vi "Mem_exper.vi"() -> ()   [LabVIEW 2018]
uses:
  <vilib>/Platform/TimedLoop/XDataNode/timing_clust.ctl
  <vilib>/Platform/TimedLoop/XDataNode/nitl_modes.ctl
  <vilib>/Platform/TimedLoop/XDataNode/wakeup.ctl
  <vilib>/rvi/eio/common/nirviEmuTemplateMethod_errors.vi
  <vilib>/rvi/Emulation/niFpgaGetClockAttributes.vi
  <vilib>/rvi/Emulation/niFpgaSctlEmulationGetInTimedLoop.vi
  <vilib>/rvi/Emulation/niFpgaEmulationReportErrorSimple.vi
  <vilib>/rvi/Emulation/niFpgaCriticalErrorInLSC.vi
  <vilib>/rvi/Memory/Memory_Emulation/niFpgaMemoryFastEmulationDramWriteAndRequestData.vi
  <vilib>/rvi/Memory/Memory_Emulation/niFpgaMemoryEmulationDramWriteAndRequestData.vi
  <vilib>/rvi/DataTransferAndStorage/Container/Common/niFpgaContainerGetUniqueNameForEmu.vi
  <vilib>/rvi/Memory/Memory_Emulation/niFpgaMemoryEmulationDramWriteAndRequestDataApplyByteEnables.vi
  <vilib>/rvi/Emulation/niFpgaProcessEmulError.vi
  <vilib>/eio/EIONode/EIONode.xnode
  <vilib>/Platform/TimedLoop/XDataNode/XDataNode.xnode
  <vilib>/rvi/DataTransferAndStorage/Container/XNode/niFpgaContainer.xnode
  <vilib>/rvi/Memory/Memory_Emulation/niFpgaMemoryEmulationDramRetrieveData.vi
  <vilib>/Platform/TimedLoop/XDataNode/XDNodeRunTimeDep.lvlib
panel:
  in  "512":u16=512
  out "Записали FIFO":bool
  in  "Кон_адр":u32=81920
  in  "Нач_адр":u32
  in  "Кадр в ПЛИС":bool
  in  "641":u16=641
  in  "514":u16=514
  in  "650":u16=650
  in  "СТОП!":bool
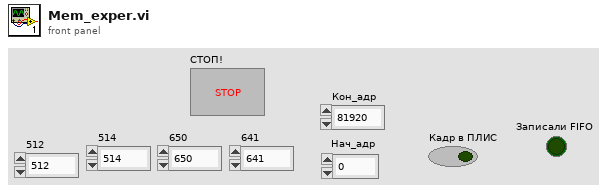
[diagram p1: front panel]
types:
  T1 = typedef "XDNodeRunTimeDep.lvlib/timing_clust.ctl" = cluster{"Expected End [f-1]":u64, "Actual End [f-1]":u64, "Finished Late? [f-1]":bool, "Expected End [i-1]":u64, "Actual End [i-1]":u64, "Finished Late? [i-1]":bool, "Expected Start [i]":u64, "Actual Start [i]":u64, "Expected Start [f]":u64, "Actual Start [f]":u64, "Source Name":string, "Structure Name":string, "Period":i64, "Deadline":i64, "Offset":i64, "Start":i64, "Priority":i32, "Timeout":i32, "Mode":T2, "Wakeup Reason":T3, "Error":errorcluster, "Source Type":string, "Secondary Source Type":string, "Global End Time":u64, "Global Start Time":u64, "Frame Duration":u64, "Iteration Duration":u64, "Assigned CPU":i32, "I/O Scan Engine Mode":u32}
  T2 = typedef "XDNodeRunTimeDep.lvlib/nitl_modes.ctl" = enum32{"No Change", "Process missed periods, maintain original phase", "Discard missed periods, maintain original phase", "Process missed periods, ignore original phase", "Discard missed periods, ignore original phase"}
  T3 = typedef "XDNodeRunTimeDep.lvlib/wakeup.ctl" = enum32{"Normal", "Aborted", "Asynchronous wakeup", "Timing source error", "Timed loop error", "Timeout"}
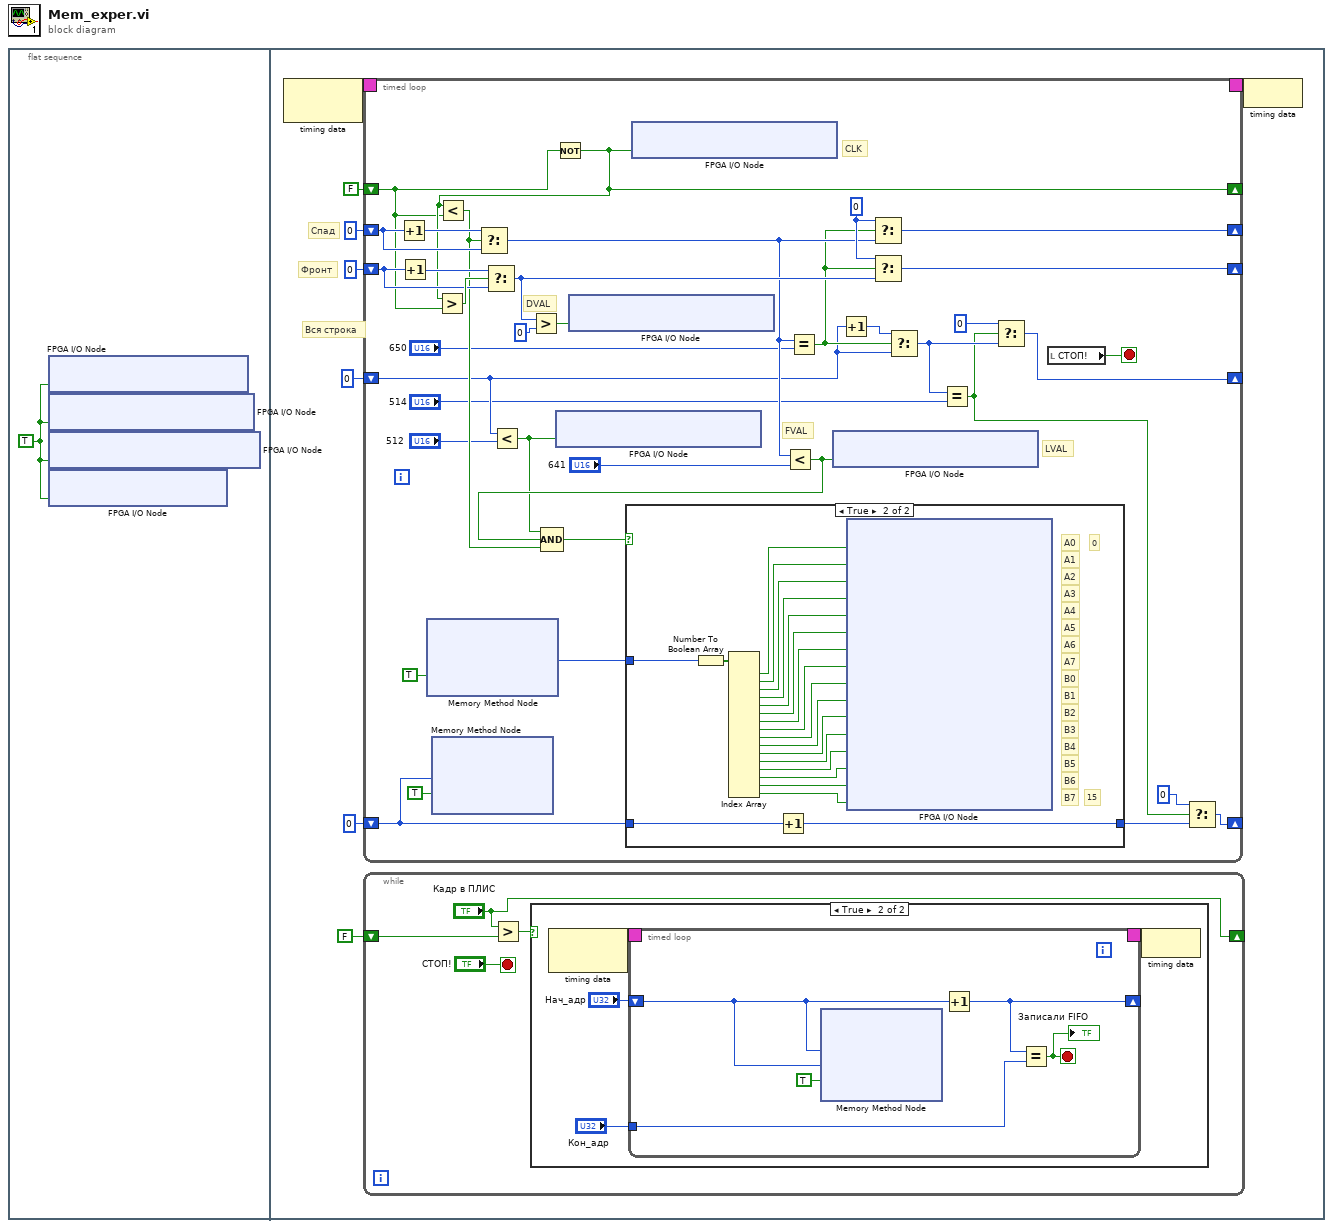
[diagram p0: block diagram]
diagram:
  n1 = flat-sequence {
    frame #0 {
      w1 = TRUE
      n2 = xnode "FPGA I/O Node"("IO Module\\DDCB_DIO0-7_WE"=w1) -> ()  [unwired: 1 in, 1 out]
      n3 = xnode "FPGA I/O Node"("IO Module\\DDCB_DIO8-15_WE"=w1) -> ()  [unwired: 1 in, 1 out]
      n4 = xnode "FPGA I/O Node"("IO Module\\DDCB_DIO16-23_WE"=w1) -> ()  [unwired: 1 in, 1 out]
      n5 = xnode "FPGA I/O Node"("IO Module\\DDCB_PFI_WE"=w1) -> ()  [unwired: 1 in, 1 out]
    }
    frame #1 {
      # "Вся строка"
      # "Фронт"
      # "Спад"
      n6 = node-c288() -> (w8:T1)  [unwired: 1 in]
      n7 = timed-loop {
        timing: w8 -> [_]
        timing-out: [_] -> w7
        shift-right: [w39] -> _
        shift-left: u16 0 -> [w45]
        shift-right: [w37] -> _
        shift-left: u16 0 -> [w42]
        shift-right: [w33] -> _
        shift-left: u16 0 -> [w24]
        shift-right: [w28] -> _
        shift-left: u32 0 -> [w20]
        shift-right: [w19] -> _
        shift-left: FALSE -> [w18]
        stop <- w10 stop-if-true
        w38 = u16 0
        # "FVAL"
        # "LVAL"
        # "DVAL"
        # "CLK"
        n8 = Increment(x=w45) -> (x+1=w46:u16)
        n9 = Increment(x=w42) -> (x+1=w43:u16)
        n10 = xnode ("Memory Method Node")("Ready for Output"=TRUE) -> ("Data"=w21:u16)  [unwired: 1 in, 2 out]
        n11 = xnode ("Memory Method Node")("Address"=w20, "Input Valid"=TRUE) -> ()  [unwired: 1 in, 2 out]
        n12 = Less?(x=w24, y="512") -> (x < y?=w23:bool)
        n13 = Not(x=w18) -> (.not. x?=w19:bool)
        n14 = Greater?(x=w19, y=w18) -> (0:w44:bool)
        n15 = Less?(x=w19, y=w18) -> (x < y?=w31:bool)
        n16 = Select(t=w46, s=w31, f=w45) -> (s? t:f=w32:u16)
        n17 = Select(t=w43, s=w44, f=w42) -> (s? t:f=w36:u16)
        n18 = Greater?(x=w36, y=u16 0) -> (0:w40:bool)
        n19 = xnode "FPGA I/O Node"("IO Module\\DDCB_DIO15_Write"=w23) -> ()  [unwired: 1 in, 1 out]
        n20 = xnode "FPGA I/O Node"("IO Module\\DDCB_DIO22_Write"=w40) -> ()  [unwired: 1 in, 1 out]
        n21 = xnode "FPGA I/O Node"("IO Module\\DDCB_DIO23_Write"=w19) -> ()  [unwired: 1 in, 1 out]
        n22 = Less?(x=w32, y="641") -> (x < y?=w30:bool)
        n23 = Compound Arithmetic op=AND(w23, w30, w31) -> (w29:bool)
        n24 = case shown="True" w29 {
          tunnel: w20 -> [w47 w48]
          tunnel: [w47 w50] -> w27
          tunnel: w21 -> [_ w49]
          frame False {
          }
          frame True {
            # "15"
            # "0"
            # "B7"
            # "B6"
            # "B5"
            # "B4"
            # "B3"
            # "B2"
            # "B1"
            # "B0"
            # "A7"
            # "A6"
            # "А5"
            # "А4"
            # "А3"
            # "А2"
            # "А1"
            # "А0"
            n25 = Number To Boolean Array(number=w49) -> (Boolean array=w67:bool[])
            n26 = Index Array(array=w67) -> (element #1=w66:bool, element #2=w65:bool, element #3=w64:bool, element #4=w63:bool, element #5=w62:bool, element #6=w61:bool, element #7=w60:bool, element #8=w59:bool, element #9=w58:bool, element #10=w57:bool, element #11=w56:bool, element #12=w55:bool, element #13=w54:bool, element #14=w53:bool, element #15=w52:bool, element #16=w51:bool)  [unwired: 16 in]
            n27 = Increment(x=w48) -> (x+1=w50:u32)
            n28 = xnode "FPGA I/O Node"("IO Module\\DDCB_DIO20_Write"=w66, "IO Module\\DDCB_DIO19_Write"=w65, "IO Module\\DDCB_DIO18_Write"=w64, "IO Module\\DDCB_DIO17_Write"=w63, "IO Module\\DDCB_DIO16_Write"=w62, "IO Module\\DDCB_PFI2_Write"=w61, "IO Module\\DDCB_DIO21_Write"=w60, "IO Module\\DDCB_PFI1_Write"=w59, "IO Module\\DDCB_PFI3_Write"=w58, "IO Module\\DDCB_DIO0_Write"=w57, "IO Module\\DDCB_DIO1_Write"=w56, "IO Module\\DDCB_DIO4_Write"=w55, "IO Module\\DDCB_DIO5_Write"=w54, "IO Module\\DDCB_DIO6_Write"=w53, "IO Module\\DDCB_DIO2_Write"=w52, "IO Module\\DDCB_DIO3_Write"=w51) -> ()  [unwired: 16 in, 16 out]
          }
        }
        n29 = Equal?(x=w32, y="650") -> (x = y?=w25:bool)
        n30 = xnode "FPGA I/O Node"("IO Module\\DDCB_DIO14_Write"=w30) -> ()  [unwired: 1 in, 1 out]
        n31 = Increment(x=w24) -> (x+1=w35:u16)
        n32 = Select(t=w38, s=w25, f=w32) -> (s? t:f=w39:u16)
        n33 = Select(t=w38, s=w25, f=w36) -> (s? t:f=w37:u16)
        n34 = Select(t=w35, s=w25, f=w24) -> (s? t:f=w22:u16)
        n35 = Equal?(x=w22, y="514") -> (x = y?=w11:bool)
        n36 = Select(t=u16 0, s=w11, f=w22) -> (s? t:f=w33:u16)
        n37 = local read "СТОП!"() -> (w10:bool)
        n38 = Select(t=u32 0, s=w11, f=w27) -> (s? t:f=w28:u32)
      }
      n39 = while {
        shift-right: ["Кадр в ПЛИС"] -> _
        shift-left: FALSE ("Кадр в ПЛИС") -> [w75]
        stop <- "СТОП!" stop-if-true
        n40 = Greater?(x="Кадр в ПЛИС", y=w75) -> (0:w73:bool)
        n41 = case shown="True" w73 {
          frame False {
          }
          frame True {
            n42 = node-c288() -> (w79:T1)  [unwired: 1 in]
            n43 = timed-loop {
              timing: w79 -> [_]
              timing-out: [_] -> w78
              shift-right: [w84] -> _
              shift-left: "Нач_адр" -> [w80]
              tunnel: "Кон_адр" -> [w82]
              stop <- w83 stop-if-true
              n44 = xnode ("Memory Method Node")("Address"=w80, "Data"=w80, "Input Valid"=TRUE) -> ()  [unwired: 1 in, 2 out]
              n45 = Increment(x=w80) -> (x+1=w84:u32)
              n46 = Equal?(x=w84, y=w82) -> (x = y?=w83:bool)
              "Записали FIFO" <- w83
            }
            n47 = node-c288(w78) -> ()
          }
        }
      }
      n48 = node-c288(w7) -> ()
    }
  }
